vi "forvard movie.vi"() -> ()   [LabVIEW 2012, in "LightPipes.lvlib"]
uses:
  LightPipes.lvlib
panel:
  in  "Set Value":dbl
  in  "Inc Step":dbl=0.0001
  out "Value":dbl
  out "Intensity":dbl[][](graph) caption="Distance: 0.00000"
  in  "Source Intensity":path=path "C:/Users/Tri/Documents/Lightpipes/LabView/data4/retrieved_target_int.dat"
  in  "stop":bool
  out "Wave Front":dbl[][](graph) caption="Distance: 0.00000"
  in  "Source Phase":path=path "C:/Users/Tri/Documents/Lightpipes/LabView/data4/retrieved_target_phase.dat"
  in  "lambda":dbl=1.054e-06
  in  "size_grid":dbl=0.001776
  in  "n_grid":i32=300
  in  "Forward Distance":dbl(slide) step=0.0001 scale=-0.02..0.02
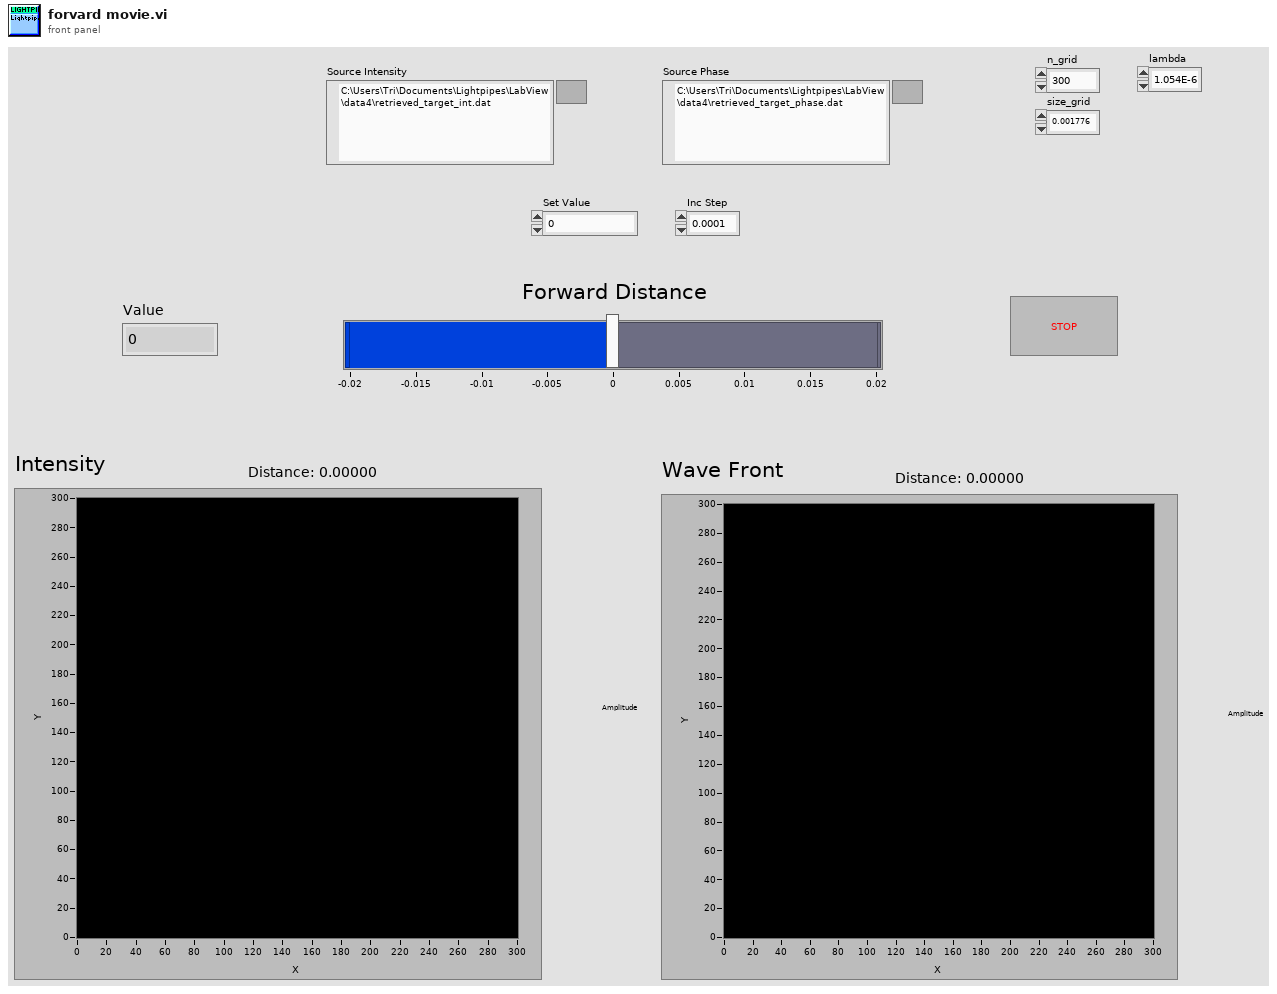
[diagram p1: front panel]
types:
  T1 = cluster{"n_grid":i32, "@dummy control@":i8, "@dummy control@":i8, "@dummy control@":i8, "@dummy control@":i8, "size":dbl, "lambda":dbl, "int1":i32, "int2":i32, "int3":i32, "@dummy control@":i8, "@dummy control@":i8, "@dummy control@":i8, "@dummy control@":i8, "double1":dbl, "double2":dbl, "double3":dbl, "real":u32, "imaginary":u32}
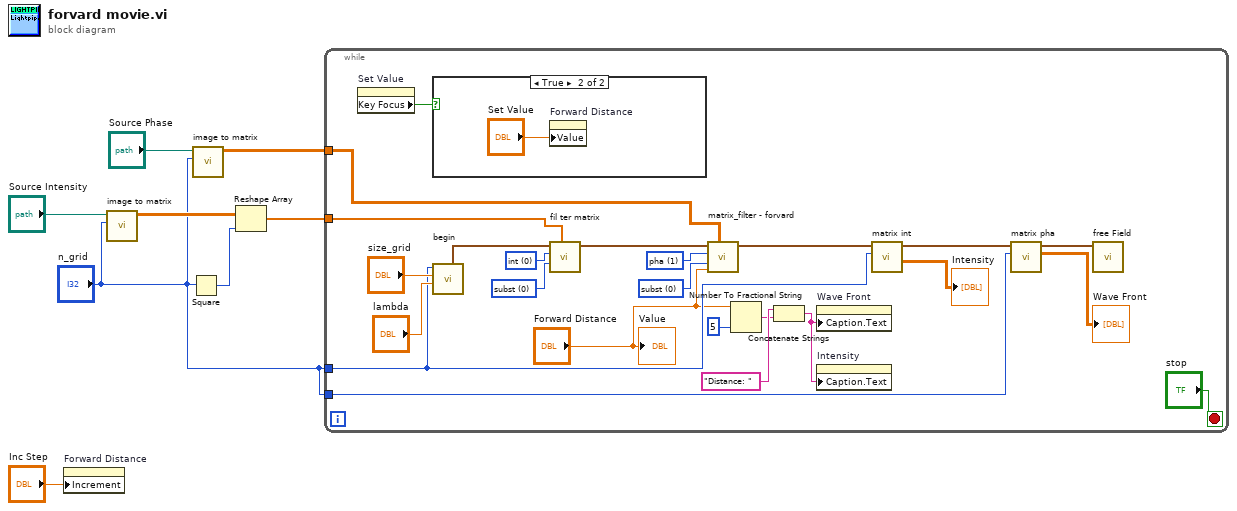
[diagram p0: block diagram]
diagram:
  n1 = property on="Forward Distance" class="Slide (strict)"("Increment"="Inc Step") -> ()  [unwired: 2 in, 2 out]
  n2 = call "image to matrix.vi"("matrixSize"="n_grid", "Image Path"="Source Intensity") -> ("matrix out 2D"=w5:dbl[][])  [unwired: 9 in]
  n3 = Square(x="n_grid") -> (x^2=w2:i32)
  n4 = call "image to matrix.vi"("matrixSize"="n_grid", "Image Path"="Source Phase") -> ("matrix out 2D"=w8:dbl[][])  [unwired: 9 in]
  n5 = Reshape Array "Reshape Array"(w5, w2) -> (w4:dbl[])
  n6 = while {
    tunnel: "n_grid" -> [w14]
    tunnel: "n_grid" -> [w26]
    tunnel: w8 -> [w25]
    tunnel: w4 -> [w17]
    stop <- "stop" stop-if-true
    w29 = i16 0 items=["subst", "mult"] ("multiplication/ substitution")
    w30 = i16 1 items=["int", "pha"] ("intensity / phase")
    w18 = i16 0 items=["int", "pha"] ("intensity / phase")
    w19 = i16 0 items=["subst", "mult"] ("multiplication/ substitution")
    n7 = property on="Set Value" class="DigNum (strict)"() -> ("Key Focus"=w9:bool)  [unwired: 2 in, 2 out]
    n8 = case shown="True" w9 {
      frame False {
      }
      frame True {
        n9 = property on="Forward Distance" class="Slide (strict)"("Value"="Set Value") -> ()  [unwired: 2 in, 2 out]
      }
    }
    n10 = call "begin.vi"("lambda"="lambda", "size_grid"="size_grid", "n_grid"=w14) -> ("field out"=w21:T1)  [unwired: 8 in]
    n11 = call "fil ter matrix.vi"("matrix"=w17, "multiplication/ substitution"=w19, "intensity / phase"=w18, "field"=w21) -> ("field out"=w20:T1)  [unwired: 6 in, 1 out]
    n12 = call "matrix_filter - forvard.vi"("matrix in"=w25, "forward distance"="Forward Distance", "multiplication/substitution"=w29, "intensity/phase"=w30, "field"=w20) -> ("field out"=w16:T1)  [unwired: 5 in, 1 out]
    n13 = Number To Fractional String(number="Forward Distance", precision (6)=i16 5 ("width (-)")) -> (F-format string=w22:string)  [unwired: 2 in]
    n14 = Concatenate Strings("Distance: " ("string"), w22) -> (w10:string)
    n15 = property on="Wave Front" class="IntGraph (strict)"("Caption.Text"=w10) -> ()  [unwired: 2 in, 2 out]
    n16 = property on="Intensity" class="IntGraph (strict)"("Caption.Text"=w10) -> ()  [unwired: 2 in, 2 out]
    n17 = call "matrix int.vi"("n_grid"=w14, "field"=w16) -> ("matrix out 2D"=→"Intensity":dbl[][], "field out"=w15:T1)  [unwired: 8 in]
    n18 = call "matrix pha.vi"("n_grid"=w26, "field"=w15) -> ("matrix out 2D"=→"Wave Front":dbl[][], "field out"=w24:T1)  [unwired: 8 in]
    n19 = call "free Field.vi"("field"=w24) -> ()  [unwired: 10 in, 1 out]
    "Value" <- "Forward Distance"
  }
